vi "convertand save to array(SubVI).vi"(10 "read buffer":string, 11 "read buffer 2":string) -> (2 "Array 2":u32[](array[numeric]), 3 "Array":u32[](array[numeric]))   [LabVIEW 2015]
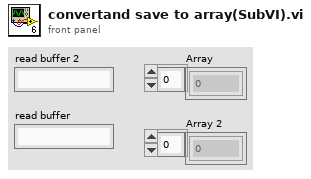
[diagram p1: front panel]
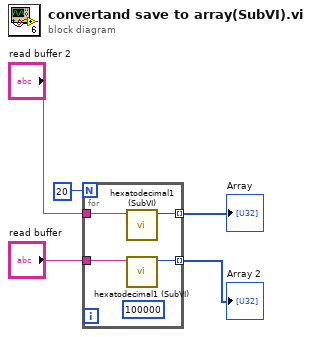
[diagram p0: block diagram]
diagram:
  n1 = for {
    N: 20 -> [_]
    tunnel: "read buffer 2" -> [w9]
    tunnel: "read buffer" -> [w8]
    tunnel: [w7] -> w5 mode=indexing
    tunnel: [w6] -> w4 mode=indexing
    (unwired) u32 100000 ("y")
    n2 = call "hexatodecimal1 (SubVI).vi"("string in"=w9) -> ("Numeric"=w7:u32)  [unwired: 10 in]
    n3 = call "hexatodecimal1 (SubVI).vi"("string in"=w8) -> ("Numeric"=w6:u32)  [unwired: 10 in]
  }
  "Array" <- w5
  "Array 2" <- w4
